vi "EOL Initialize All Inputs And ErrorHandler.vi"(8 "Sys Error In":errorcluster, 10 "DI Map Path":path=path "C:/Labview Code/System/Digital Input Channel Configuration", 11 "Error Table Path":path=path "C:/Labview Code/System/Error Table") -> (0 "Sys Error Out":errorcluster)   [LabVIEW 2018]
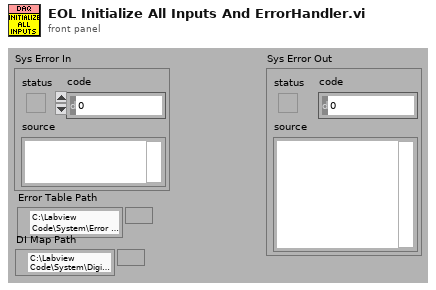
[diagram p1: front panel]
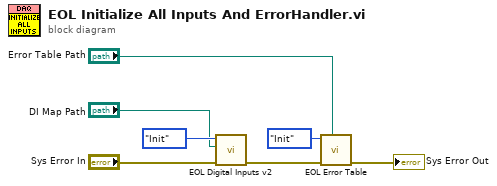
[diagram p0: block diagram]
diagram:
  n1 = call "EOL Digital Inputs v2.vi"("Sys Error In"="Sys Error In", "DI Map path"="DI Map Path", "Mode"=enum16{"Init", "Read", "Read All", "Close"}."Init") -> ("Sys Error Out"=w1:errorcluster)  [unwired: 6 in, 2 out]
  n2 = call "EOL Error Table.vi"("Path"="Error Table Path", "error in"=w1, "Error Mode"=enum16{"Init", "Get Error"}."Init") -> ("error out"=→"Sys Error Out":errorcluster)  [unwired: 7 in, 1 out]
